vi "Transport.vi"(7 "Actor in":refnum<class "Actor.lvclass">) -> (2 "Transport":refnum<class "Transport.lvclass">)   [LabVIEW 2020, in "jettl.lvlib" / "Read Self Attributes.lvlib"]
uses:
  Read Self Attributes.lvlib
  Actor/Actor.lvclass
  Transport/Transport.lvclass
  Attributes/Attributes.lvclass
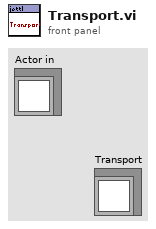
[diagram p1: front panel]
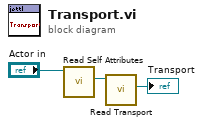
[diagram p0: block diagram]
diagram:
  n1 = call-dynamic "Read Self Attributes.vi"("Actor in"="Actor in") -> ("Self Attributes"=w2:refnum<class "Attributes.lvclass">)  [unwired: 10 in]
  n2 = call-dynamic "Read Transport.vi"("Attributes in"=w2) -> ("Transport"=→"Transport":refnum<class "Transport.lvclass">)  [unwired: 10 in]
